vi "Get_User_Limit.vi"(8 "error in":errorcluster, 11 "VISA name":refnum<visa-resource-name>) -> (0 "error out":errorcluster, 1 "valid":bool, 2 "UserLimit /Ohms":dbl, 3 "VISA out":refnum<visa-resource-name>)   [LabVIEW 2023, in "QR 10X Eastwood.lvlib"]
uses:
  <instrlib>/QR 10X Eastwood/QR 10X Eastwood.lvlib
panel:
  out "buffer":string
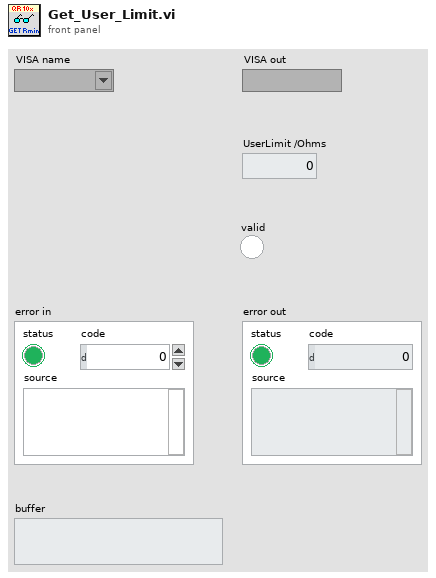
[diagram p1: front panel]
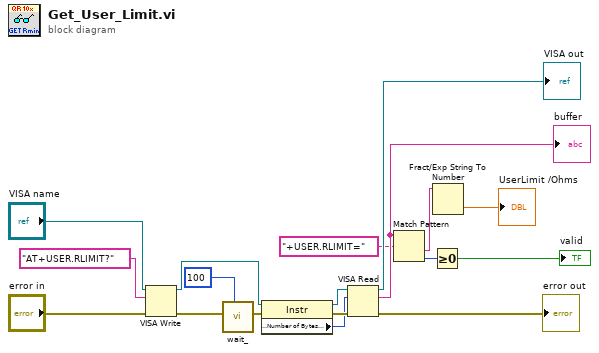
[diagram p0: block diagram]
diagram:
  n1 = VISA Write(VISA resource name="VISA name", write buffer="AT+USER.RLIMIT?", error in (no error)="error in") -> (VISA resource name out=w17:refnum<visa-resource-name>, error out=w3:errorcluster)  [unwired: 1 out]
  n2 = call "wait_.vi"("milliseconds to wait"=u32 100, "error in"=w3) -> ("error out"=w2:errorcluster)  [unwired: 9 in]
  n3 = property class="Instr"(reference=w17, error in=w2) -> (reference out=w16:refnum<visa-resource-name>, error out=w15:errorcluster, "Serial Settings:Number of Bytes at Serial Port"=w14:u32)
  n4 = VISA Read(VISA resource name=w16, byte count=w14, error in (no error)=w15) -> (VISA resource name out=→"VISA out":refnum<visa-resource-name>, read buffer=w8:string, error out=→"error out":errorcluster)  [unwired: 1 out]
  "buffer" <- w8
  n5 = Match Pattern(string=w8, regular expression="+USER.RLIMIT=") -> (after substring=w6:string, offset past match=w5:i32)  [unwired: 1 in, 2 out]
  n6 = Greater Or Equal To 0?(x=w5) -> (x >= 0?=→"valid":bool)
  n7 = Fract/Exp String To Number(string=w6) -> (number=→"UserLimit /Ohms":dbl)  [unwired: 3 in, 1 out]
